vi "Handle State Name Change.vi"(8 "error in (no error)":errorcluster, 9 "Old State Name":string, 10 "New State Name":string, 11 "Routing Channel Ref in":T1 format="%.0x") -> (0 "error out":errorcluster, 1 "State to Display":string, 3 "Routing Channel Ref out":T1 format="%.0x")   [LabVIEW 2020, in "Routing and Faulting System Explorer.lvlib"]
uses:
  Routing and Faulting System Explorer.lvlib
  <vilib>/NI VeriStand/Custom Device API/Custom Device Item Ref.ctl
  Scripting/Routing and Faulting Scripting.lvlib
  <vilib>/NI VeriStand/Custom Device API/Custom Device API.lvlib
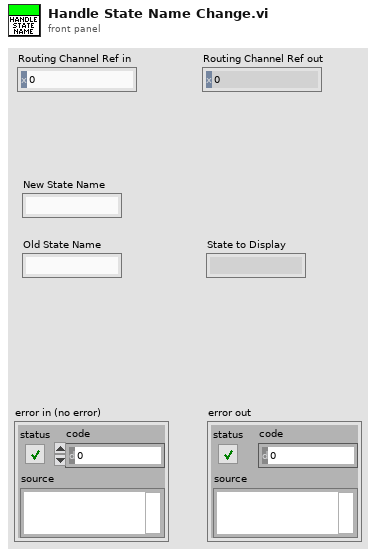
[diagram p1: front panel]
types:
  T1 = typedef "Custom Device API.lvlib/Custom Device Item Ref.ctl" = u64
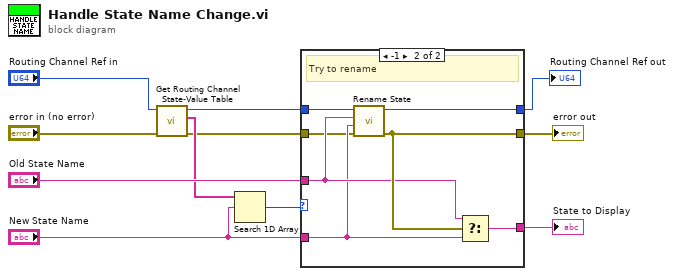
[diagram p0: block diagram]
diagram:
  n1 = call "Get Routing Channel State-Value Table.vi"("error in"="error in (no error)", "routing channel in"="Routing Channel Ref in") -> ("error out"=w2:errorcluster, "state names"=w7:string[], "routing channel out"=w3:T1)  [unwired: 6 in, 1 out]
  n2 = Search 1D Array(1D array=w7, element="New State Name") -> (index of element=w1:i32)  [unwired: 1 in]
  n3 = case shown="-1" w1 {
    tunnel: [w12 w21] -> w11
    tunnel: [w13 w20] -> w10
    tunnel: "Old State Name" -> [_ w19]
    tunnel: [w14 w18] -> w8
    tunnel: "New State Name" -> [w14 w17]
    tunnel: w3 -> [w12 w16]
    tunnel: w2 -> [w13 w15]
    frame 0, Default {
      # "Not a rename\nDisplay State of New Name"
    }
    frame -1 {
      # "Try to rename"
      n4 = call "Rename State.vi"("error in"=w15, "new state"=w17, "state"=w19, "routing channel in"=w16) -> ("error out"=w20:errorcluster, "routing channel out"=w21:T1)  [unwired: 6 in]
      n5 = Select(t=w19, s=w20, f=w17) -> (s? t:f=w18:string)
    }
  }
  "error out" <- w10
  "Routing Channel Ref out" <- w11
  "State to Display" <- w8
